vi "PH_SHS_Analysis_Calibrator.get Text for Start Procedure Dialog.vi"(0 "i ref in":refnum<vi>, 5 "error in (no error)":errorcluster) -> (14 "i ref out":refnum<vi>, 17 "Dialog Start Procedure":string, 19 "error out":errorcluster)   [LabVIEW 2014, in "PH_SHS_Analysis_Calibrator.lvlib"]
doc: "This VI creates the text for the Start procedure case. The camera is asked for its attributes (which are displayed) and its serial number. The attributes and the serial number are also written to own attributes."
uses:
  PH_SHS_Analysis_Calibrator.lvlib
  PH_Basics/PH_Common/PH_Common.lvlib
  PH_Basics/PH_Img_BaseClass/PH_Img_BaseClass.lvlib
  PH_Basics/PH_Cam_BaseClass/PH_Cam_BaseClass.lvlib
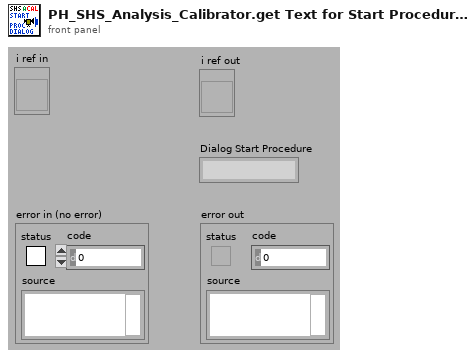
[diagram p1: front panel]
types:
  T1 = cluster{"Cam ID":string, "Gain":dbl, "Brightness":dbl, "Shutter":dbl, "Cam Error":bool, "Mode":i32}
  T2 = typedef "PH_SHS_Analysis_Calibrator.lvlib/PH_SHS_Analysis_Calibrator.i attribute.ctl" = cluster{"GUI Refs":cluster{"Available Cams":refnum<vi>, "OK":refnum<vi>, "Skip":refnum<vi>, "Repeat":refnum<vi>, "Cancel":refnum<vi>, "Dialog":refnum<vi>, "Enough Images?":refnum<vi>}, "Cam instances":string[], "Status":cluster{"#":i32, "Data calculated":bool, "Wanted #":i32}, "IMAQ Image Array":T3[], "Pixel Size [µm]":dbl, "MLA Pitch [µm]":dbl, "Method":enum16{"automatic", "manual"}, "Enough Images?":bool, "SHS Reference Result":T4, "Calculation Error":errorcluster}
  T3 = typedef "IMAQ Image.ctl" = refnum<image>
  T4 = typedef "SHS_Common.lvlib/SHSReference.ctl" = cluster{"Reference":T5[][], "Lens Array Pitch [px]":dbl}
  T5 = typedef "SHS_Common.lvlib/ReferencePoint.ctl" = cluster{"Rect":T6, "Point":T7}
  T6 = typedef "SHS_Common.lvlib/Rectangle.ctl" = cluster{"Left":i32, "Top":i32, "Right":i32, "Bottom":i32}
  T7 = typedef "SHS_Common.lvlib/Point.ctl" = cluster{"x":dbl, "y":dbl, "valid?":bool, "weight":dbl}
  T8 = typedef "PH_Img_BaseClass.lvlib/PH_Img_BaseClass.i attribute.ctl" = cluster{"GUI Refs":T9, "Timeout Image [ms]":i32, "Default Periodic Period [ms]":i32, "Camera":cluster{"Instancename":string, "Notifier":refnum<notifier>}, "Palette":T10, "Cam Settings":cluster{"Cam ID":string, "Gain":dbl, "Brightness":dbl, "Shutter":dbl, "Cam Info Failure":bool, "Mode":i32}}
  T9 = typedef "PH_Img_BaseClass.lvlib/PH_Img_BaseClass.GUI Refs.ctl" = cluster{"Timeout":refnum<vi>, "Image":refnum<vi>, "Palette":refnum<vi>, "Timeout Set":refnum<vi>}
  T10 = typedef "PH_Img_BaseClass.lvlib/PH_Img_BaseClass.Palette.ctl" = i32
  T11 = typedef "PH_Cam_BaseClass.lvlib/PH_Cam_BaseClass.Settings.ctl" = cluster{"Cam ID":string, "Gain":dbl, "Brightness":dbl, "Shutter":dbl, "Mode":i32}
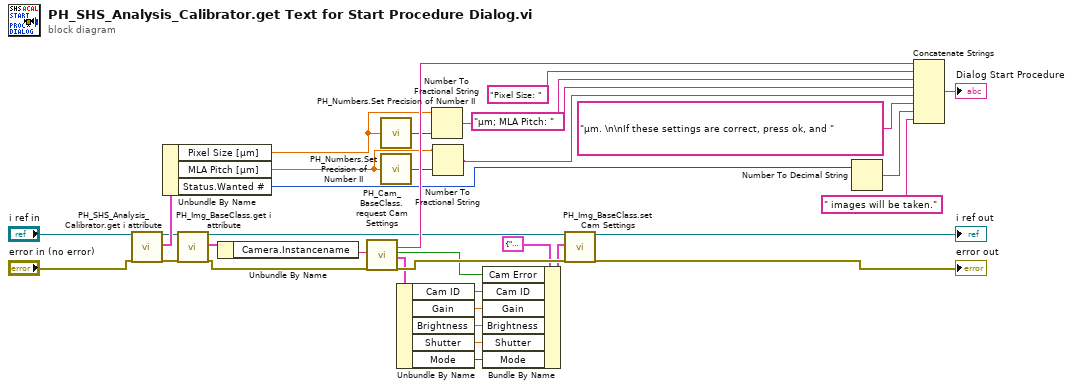
[diagram p0: block diagram]
diagram:
  n1 = call "PH_SHS_Analysis_Calibrator.get i attribute.vi"("i ref in"="i ref in", "error in (no error)"="error in (no error)") -> ("i ref out"=w27:refnum<vi>, "i attribute"=w31:T2, "error out"=w14:errorcluster)  [unwired: 15 in]
  n2 = Unbundle By Name(w31) -> ("Pixel Size [µm]"=w20:dbl, "MLA Pitch [µm]"=w17:dbl, "Status.Wanted #"=w16:i32)
  n3 = call "PH_Img_BaseClass.get i attribute.vi"("i ref in"=w27, "error in (no error)"=w14) -> ("i ref out"=w15:refnum<vi>, "i attribute"=w12:T8, "error out"=w13:errorcluster)  [unwired: 15 in]
  n4 = Unbundle By Name(w12) -> ("Camera.Instancename"=w11:string)
  n5 = call "PH_Cam_BaseClass.request Cam Settings.vi"("Cam Instance"=w11, "error in (no error)"=w13) -> ("Cam Setting Information"=w28:string, "Error getting the Data?"=w3:bool, "Cam Settings"=w29:T11, "error out"=w30:errorcluster)  [unwired: 14 in]
  n6 = call "PH_Numbers.Set Precision of Number II.vi"("Number"=w20) -> ("Precision"=w19:i32)  [unwired: 1 in]
  n7 = call "PH_Numbers.Set Precision of Number II.vi"("Number"=w17) -> ("Precision"=w18:i32)  [unwired: 1 in]
  n8 = Unbundle By Name(w29) -> ("Cam ID"=w8:string, "Gain"=w7:dbl, "Brightness"=w6:dbl, "Shutter"=w5:dbl, "Mode"=w4:i32)
  n9 = Number To Fractional String(number=w20, precision (6)=w19) -> (F-format string=w22:string)  [unwired: 2 in]
  n10 = Number To Fractional String(number=w17, precision (6)=w18) -> (F-format string=w21:string)  [unwired: 2 in]
  n11 = Bundle By Name(cluster=T1 {"Cam ID"="N/A", "Gain"=nan, "Brightness"=nan, "Shutter"=nan, "Cam Error"=TRUE, "Mode"=-1} ("Cam Settings"), "Cam Error"=w3, "Cam ID"=w8, "Gain"=w7, "Brightness"=w6, "Shutter"=w5, "Mode"=w4) -> (w1:T1)
  n12 = call "PH_Img_BaseClass.set Cam Settings.vi"("i ref in"=w15, "Cam Settings"=w1, "error in (no error)"=w30) -> ("i ref out"=→"i ref out":refnum<vi>, "error out"=→"error out":errorcluster)  [unwired: 15 in]
  n13 = Number To Decimal String(number=w16) -> (decimal integer string=w26:string)  [unwired: 1 in]
  n14 = Concatenate Strings(w28, "Pixel Size: " ("string"), w22, "µm; MLA Pitch: ", w21, "µm. \n\nIf these settings are correct, press ok, and ", w26, " images will be taken." ("string")) -> (→"Dialog Start Procedure":string)
